vi "lib Read 699 Config File.vi"(7 "Mission":string, 8 "error in (no error)":errorcluster, 10 "Write?":bool, 11 "mission folders in":T1) -> (0 "error out":errorcluster, 3 "mission folders out":T1)   [LabVIEW 2014]
uses:
  lib cluster 699 Config.ctl
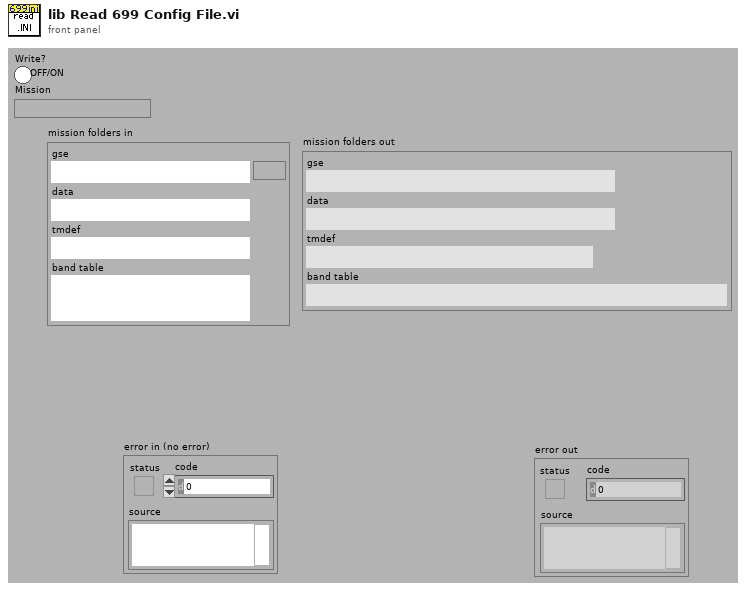
[diagram p1: front panel]
types:
  T1 = typedef "lib cluster 699 Config.ctl" = cluster{"gse":path, "data":path, "tmdef":path, "band table":path}
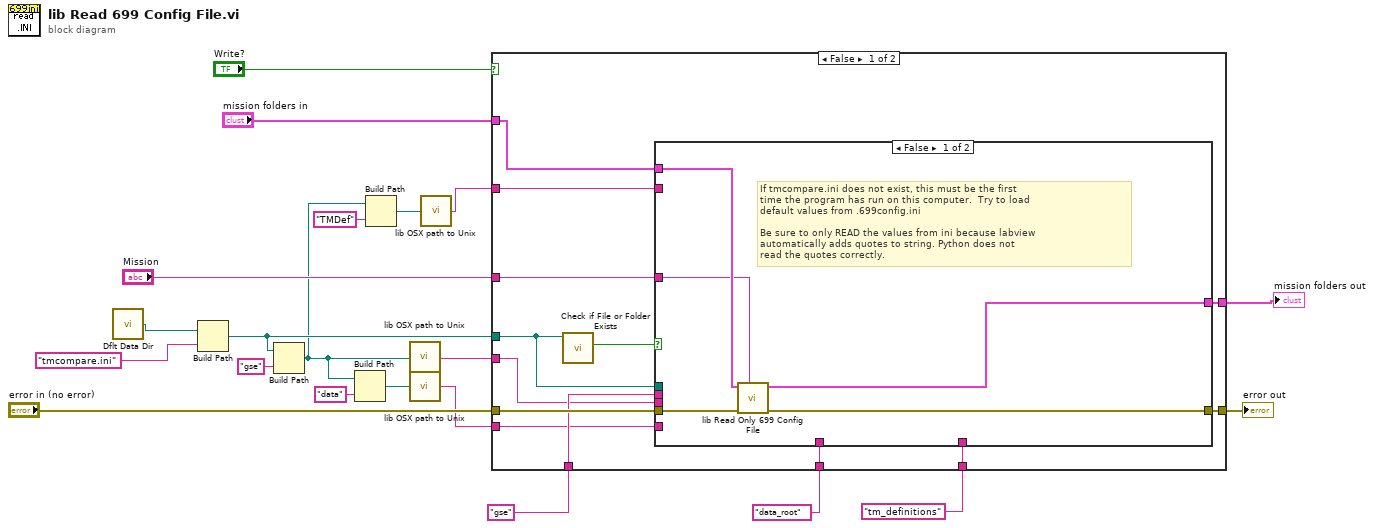
[diagram p0: block diagram]
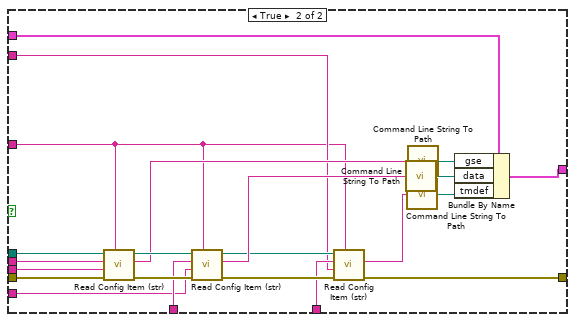
[diagram p2: hidden frame]
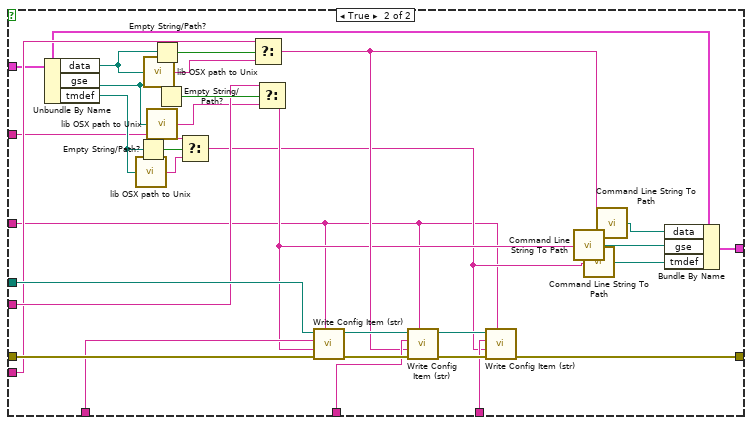
[diagram p3: hidden frame]
diagram:
  n1 = call <vilib>:"Dflt Data Dir.vi"() -> ("App:Default Data Directory"=w1:path)
  n2 = Build Path(base path=w1, name or relative path="tmcompare.ini") -> (appended path=w16:path)
  n3 = Build Path(base path=w16, name or relative path="gse") -> (appended path=w2:path)
  n4 = Build Path(base path=w2, name or relative path="data") -> (appended path=w8:path)
  n5 = Build Path(base path=w2, name or relative path="TMDef") -> (appended path=w5:path)
  n6 = call "lib OSX path to Unix.vi"("LV Path"=w2) -> ("UNIX Path"=w9:string)  [unwired: 4 in]
  n7 = call "lib OSX path to Unix.vi"("LV Path"=w8) -> ("UNIX Path"=w7:string)  [unwired: 4 in]
  n8 = call "lib OSX path to Unix.vi"("LV Path"=w5) -> ("UNIX Path"=w3:string)  [unwired: 4 in]
  n9 = case shown="False" "Write?" {
    tunnel: "error in (no error)" -> [w34 w92]
    tunnel: w16 -> [w23 w91]
    tunnel: "Mission" -> [w25 w63]
    tunnel: "gse" ("Item") -> [w33 w90]
    tunnel: w9 -> [w32 w88]
    tunnel: "data_root" ("Item") -> [w31 w83]
    tunnel: w7 -> [w30 w84]
    tunnel: [w24 w62] -> w12
    tunnel: "mission folders in" -> [w29 w82]
    tunnel: [w28 w81] -> w10
    tunnel: "tm_definitions" ("Item") -> [w27 w70]
    tunnel: w3 -> [w26 w66]
    frame False {
      n10 = call <vilib>:"Check if File or Folder Exists.vi"("path"=w23) -> ("file or folder exists?"=w22:bool)  [unwired: 8 in, 2 out]
      n11 = case shown="False" w22 {
        tunnel: w34 -> [w39 w61]
        tunnel: w33 -> [_ w60]
        tunnel: w32 -> [_ w59]
        tunnel: w31 -> [_ w56]
        tunnel: w30 -> [_ w55]
        tunnel: w29 -> [w38 w54]
        tunnel: [w36 w53] -> w28
        tunnel: w27 -> [_ w46]
        tunnel: w26 -> [_ w45]
        tunnel: w25 -> [w35 w42]
        tunnel: [w37 w41] -> w24
        tunnel: w23 -> [_ w40]
        frame False {
          # "If tmcompare.ini does not exist, this must be the first\ntime the program has run on this computer.  Try to load\ndefault values from .699config.ini\n\nBe sure to only READ the values from ini because labview\nautomatically adds quotes to string. Python does not\nread the quotes correctly."
          n12 = call "lib Read Only 699 Config File.vi"("Mission"=w35, "error in (no error)"=w39, "mission folders in"=w38) -> ("error out"=w37:errorcluster, "mission folders out"=w36:T1)  [unwired: 7 in]
        }
        frame True {
          n13 = call "Read Config Item (str).vi"("Section"=w42, "error in (no error)"=w61, "Default"=w59, "Item"=w60, "hardware configuration file path"=w40) -> ("error out"=w58:errorcluster, "Value"=w50:string, "hardware configuration file path dup"=w57:path)  [unwired: 4 in]
          n14 = call "Read Config Item (str).vi"("Section"=w42, "error in (no error)"=w58, "Default"=w55, "Item"=w56, "hardware configuration file path"=w57) -> ("error out"=w48:errorcluster, "Value"=w52:string, "hardware configuration file path dup"=w47:path)  [unwired: 4 in]
          n15 = call "Read Config Item (str).vi"("Section"=w42, "error in (no error)"=w48, "Default"=w45, "Item"=w46, "hardware configuration file path"=w47) -> ("error out"=w41:errorcluster, "Value"=w44:string)  [unwired: 4 in, 1 out]
          n16 = call <vilib>:"Command Line String To Path.vi"("string"=w52) -> ("path"=w51:path)
          n17 = call <vilib>:"Command Line String To Path.vi"("string"=w44) -> ("path"=w43:path)
          n18 = call <vilib>:"Command Line String To Path.vi"("string"=w50) -> ("path"=w49:path)
          n19 = Bundle By Name(cluster=w54, "gse"=w49, "data"=w51, "tmdef"=w43) -> (w53:T1)
        }
      }
    }
    frame True {
      n20 = Unbundle By Name(w82) -> ("data"=w78:path, "gse"=w77:path, "tmdef"=w67:path)
      n21 = call "lib OSX path to Unix.vi"("LV Path"=w67) -> ("UNIX Path"=w69:string)  [unwired: 4 in]
      n22 = Empty String/Path?(string/path=w67) -> (empty?=w68:bool)
      n23 = call "lib OSX path to Unix.vi"("LV Path"=w78) -> ("UNIX Path"=w79:string)  [unwired: 4 in]
      n24 = call "lib OSX path to Unix.vi"("LV Path"=w77) -> ("UNIX Path"=w80:string)  [unwired: 4 in]
      n25 = Empty String/Path?(string/path=w78) -> (empty?=w85:bool)
      n26 = Empty String/Path?(string/path=w77) -> (empty?=w89:bool)
      n27 = Select(t=w66, s=w68, f=w69) -> (s? t:f=w65:string)
      n28 = Select(t=w84, s=w85, f=w79) -> (s? t:f=w76:string)
      n29 = Select(t=w88, s=w89, f=w80) -> (s? t:f=w74:string)
      n30 = call "Write Config Item (str).vi"("Section"=w63, "error in (no error)"=w92, "Value"=w74, "Item"=w90, "hardware configuration file path"=w91) -> ("error out"=w87:errorcluster, "hardware configuration file path dup"=w86:path)  [unwired: 5 in]
      n31 = call "Write Config Item (str).vi"("Section"=w63, "error in (no error)"=w87, "Value"=w76, "Item"=w83, "hardware configuration file path"=w86) -> ("error out"=w72:errorcluster, "hardware configuration file path dup"=w71:path)  [unwired: 5 in]
      n32 = call "Write Config Item (str).vi"("Section"=w63, "error in (no error)"=w72, "Value"=w65, "Item"=w70, "hardware configuration file path"=w71) -> ("error out"=w62:errorcluster)  [unwired: 5 in, 1 out]
      n33 = call <vilib>:"Command Line String To Path.vi"("string"=w74) -> ("path"=w73:path)
      n34 = call <vilib>:"Command Line String To Path.vi"("string"=w65) -> ("path"=w64:path)
      n35 = call <vilib>:"Command Line String To Path.vi"("string"=w76) -> ("path"=w75:path)
      n36 = Bundle By Name(cluster=w82, "data"=w75, "gse"=w73, "tmdef"=w64) -> (w81:T1)
    }
  }
  "error out" <- w12
  "mission folders out" <- w10
